vi "MNK_FP to PGSQL.vi"(8 "error in (no error)":errorcluster, 10 "str":string[](array[string]), 11 "dbl":dbl[](array[numeric])) -> (0 "error out":errorcluster)   [LabVIEW 2013]
uses:
  postgreSQL-lv/Data.PG/Data.PGSQL.lvclass
panel:
  # "MNK FP to PGSQL"
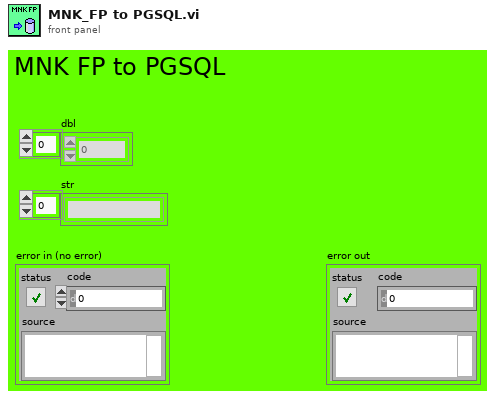
[diagram p1: front panel]
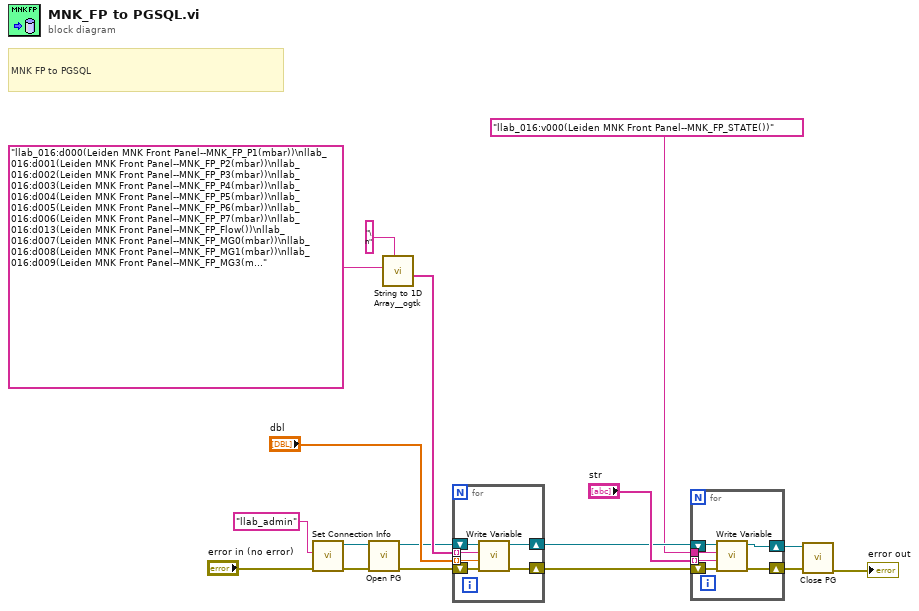
[diagram p0: block diagram]
diagram:
  # "MNK FP to PGSQL"
  n1 = call "Set Connection Info.vi"("username"="llab_admin", "error in (no error)"="error in (no error)") -> ("Data.PG out"=w2:refnum<class "Data.PGSQL.lvclass">, "error out"=w3:errorcluster)  [unwired: 7 in]
  n2 = call-dynamic "Open PG.vi"("error in (no error)"=w3, "Data.PG in"=w2) -> ("error out"=w4:errorcluster, "Data.PG out"=w1:refnum<class "Data.PGSQL.lvclass">)  [unwired: 8 in]
  n3 = call <userlib>:"String to 1D Array__ogtk.vi"("delimiter (Tab)"="\n", "string"="llab_016:d000(Leiden MNK Front Panel--MNK_FP_P1(mbar))\nllab_016:d001(Leiden MNK Front Panel--MNK_FP_P2(mbar))\nllab_016:d002(Leiden MNK Front Panel--MNK_FP_P3(mbar))\nllab_016:d003(Leiden MNK Front Panel--MNK_FP_P4(mbar))\nllab_016:d004(Leiden MNK Front Panel--MNK_FP_P5(mbar))\nllab_016:d005(Leiden MNK Front Panel--MNK_FP_P6(mbar))\nllab_016:d006(Leiden MNK Front Panel--MNK_FP_P7(mbar))\nllab_016:d013(Leiden MNK Front Panel--MNK_FP_Flow())\nllab_016:d007(Leiden MNK Front Panel--MNK_FP_MG0(mbar))\nllab_016:d008(Leiden MNK Front Panel--MNK_FP_MG1(mbar))\nllab_016:d009(Leiden MNK Front Panel--MNK_FP_MG3(mbar))\nllab_016:d010(Leiden MNK Front Panel--MNK_FP_MG4(mbar))\nllab_016:d011(Leiden MNK Front Panel--MNK_FP_MG5(mbar))\nllab_016:d014(Leiden MNK Front Panel--MNK_FP_state0())\nllab_016:d015(Leiden MNK Front Panel--MNK_FP_state1())\nllab_016:d016(Leiden MNK Front Panel--MNK_FP_state2())") -> ("Array of Strings"=w13:string[])  [unwired: 9 in]
  n4 = for {
    tunnel: w13 -> [w21] mode=indexing
    tunnel: "dbl" -> [w18] mode=indexing
    shift-right: [w19] -> w10
    shift-left: w1 -> [w22]
    shift-right: [w20] -> w9
    shift-left: w4 -> [w23]
    n5 = call "Write Variable.vi"("error in (no error)"=w23, "Data"=w18, "variable"=w21, "Data.PG in"=w22) -> ("error out"=w20:errorcluster, "Data.PG out"=w19:refnum<class "Data.PGSQL.lvclass">)  [unwired: 5 in, 1 out]
  }
  n6 = for {
    tunnel: "llab_016:v000(Leiden MNK Front Panel--MNK_FP_STATE())" -> [w26]
    tunnel: "str" -> [w25] mode=indexing
    shift-right: [w24] -> w5
    shift-left: w10 -> [w28]
    shift-right: [w27] -> w7
    shift-left: w9 -> [w29]
    n7 = call "Write Variable.vi"("error in (no error)"=w29, "Data"=w25, "variable"=w26, "Data.PG in"=w28) -> ("error out"=w27:errorcluster, "Data.PG out"=w24:refnum<class "Data.PGSQL.lvclass">)  [unwired: 5 in, 1 out]
  }
  n8 = call-dynamic "Close PG.vi"("error in (no error)"=w7, "Data.PG in"=w5) -> ("error out"=→"error out":errorcluster)  [unwired: 8 in, 1 out]
